vi "CRYData View Graph Set.vi"(9 "Title State":bool, 10 "Flattened Graph ViewPro":string, 11 "Queue Name":string) -> ()   [LabVIEW 2013]
uses:
  CRYData View Global.vi
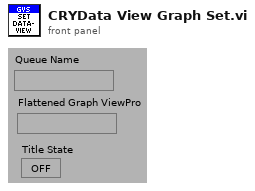
[diagram p1: front panel]
types:
  T1 = typedef "CRYGraph Property.ctl" = cluster{"LegendShow":bool, "Legend Splitter Position":dbl, "Data Names":string[], "Item Symbols":i32[], "Color Array":u32[], "Flattened Plot Property":string, "CursorShow":bool, "Flattened Cursor Property":string, "Graph Number":i32, "Flattened Scale Property":string, "PreviewShow":bool, "MagnitudeShow":bool, "PaletteShow":bool, "XYShow":bool, "FrequencyShow":bool, "Frequency Splitter Position":dbl, "XYGraph Splitter Position":dbl, "Frequency Symbols":i32[], "LegendVScrollShow":bool, "FrequencyVScrollShow":bool, "PhaseShow":bool, "Title Name":string}
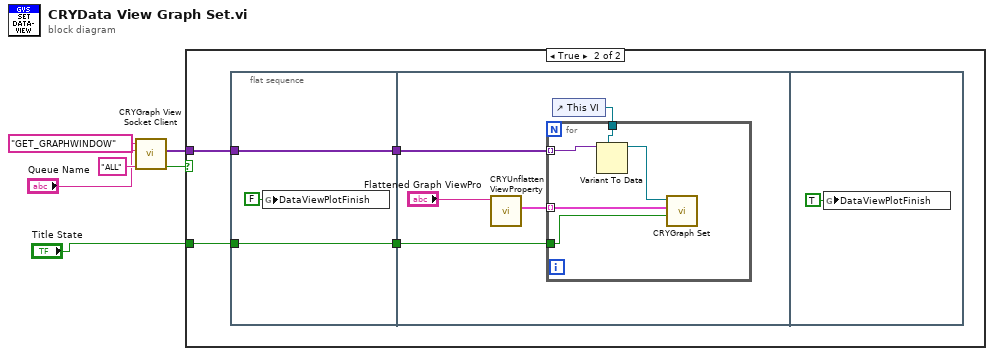
[diagram p0: block diagram]
diagram:
  n1 = call "CRYGraph View Socket Client.vi"("sOption"="ALL", "sData"="Queue Name", "sAction"="GET_GRAPHWINDOW") -> ("bResult Out"=w2:bool, "Variant Out"=w3:variant[])  [unwired: 5 in, 2 out]
  n2 = case shown="True" w2 {
    tunnel: w3 -> [_ w10]
    tunnel: "Title State" -> [_ w7]
    frame False {
    }
    frame True {
      n3 = flat-sequence {
        tunnel: w10 -> [w13]
        tunnel: [w13] -> w9
        tunnel: [w11] -> w8
        tunnel: w7 -> [w11]
        tunnel: w9 -> [w18]
        tunnel: w8 -> [w14]
        frame #0 {
          n4 = global write "CRYData View Global.vi" "DataViewPlotFinish"(FALSE ("DataViewPlotFinish")) -> ()
        }
        frame #1 {
          n5 = call "CRYUnflatten ViewProperty.vi"("Flatten ViewPro"="Flattened Graph ViewPro") -> ("ViewPro Cluster"=w16:T1[])  [unwired: 8 in, 2 out]
          n6 = control-ref of="This VI"() -> (w15:refnum<vi>)
          n7 = for {
            tunnel: w16 -> [w19] mode=indexing
            tunnel: w18 -> [w23] mode=indexing
            tunnel: w15 -> [w22]
            tunnel: w14 -> [w20]
            n8 = Variant To Data(type=w22, Variant=w23) -> (data=w21:refnum<vi>)  [unwired: 1 in, 1 out]
            n9 = call "CRYGraph Set.vi"("Title State"=w20, "Graph Property"=w19, "pGraph VI In"=w21) -> ()  [unwired: 9 in]
          }
        }
        frame #2 {
          n10 = global write "CRYData View Global.vi" "DataViewPlotFinish"(TRUE ("DataViewPlotFinish")) -> ()
        }
      }
    }
  }
